vi "qODC.vi"(0 "System no.":i32=1 min=1 max=4 step=1, 2 "Axes to query":string[](array[string]), 3 "All axes?":bool, 4 "Axis identifier?":bool=TRUE, 5 "error in":errorcluster) -> (14 "Deceleration":dbl[](array[numeric]) format="%.6f", 19 "error out":errorcluster)   [LabVIEW 2020]
doc: "Returns open-loop deceleration setting for specified axes.\n\nE-861, E-874: If All axes? = TRUE, then Axis identifier? can be FALSE. Deceleration unit is steps/s²."
panel:
  # "Returns open-loop deceleration setting for specified axes."
  # "If all axes: use"
  # "Query"
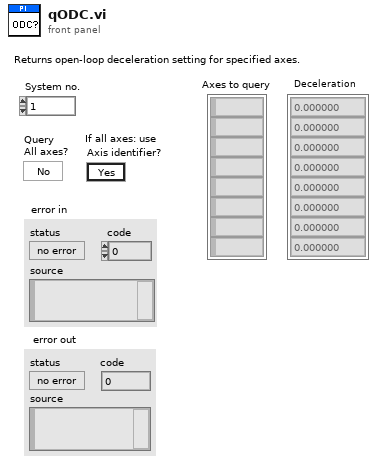
[diagram p1: front panel]
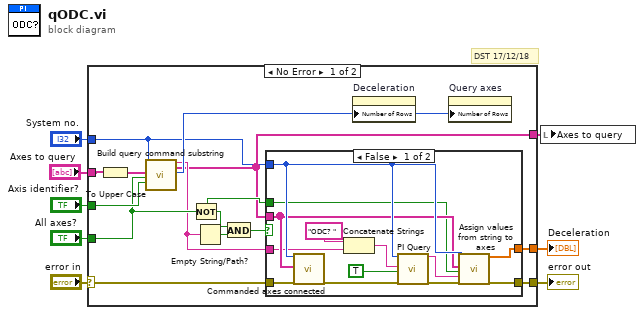
[diagram p0: block diagram]
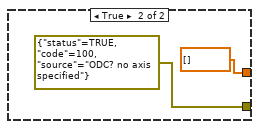
[diagram p2: hidden frame]
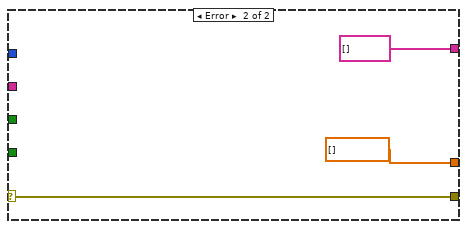
[diagram p3: hidden frame]
diagram:
  # "DST 17/12/18"
  n1 = case shown="No Error" "error in" {
    selector: "error in" -> [w10 w38]
    tunnel: [w22 dbl[] [] ("Values")] -> w8
    tunnel: "Axes to query" -> [w21 _]
    tunnel: [w20 w38] -> w6
    tunnel: "Axis identifier?" -> [w18 _]
    tunnel: "System no." -> [w16 _]
    tunnel: "All axes?" -> [w15 _]
    tunnel: [w9 string[] [] ("Axes to query out")] -> w1
    frame No Error {
      n2 = To Upper Case(1:w21) -> (0:w19:string[])
      n3 = call "Build query command substring.vi"("System no."=w16, "Axes to query in"=w19, "Query\nAll axes?"=w15, "For all axes: use\nAxis identifier?"=w18) -> ("Command substring"=w13:string, "Axes to query out"=w9:string[], "Number of rows"=w17:u32)  [unwired: 2 in, 11 out]
      n4 = Not(x=w15) -> (.not. x?=w14:bool)
      n5 = Empty String/Path?(string/path=w13) -> (empty?=w12:bool)
      n6 = And(x=w14, y=w12) -> (x .and. y?=w11:bool)
      n7 = case shown="False" w11 {
        tunnel: [w32 dbl[] [] ("Values")] -> w22
        tunnel: w10 -> [w31 _]
        tunnel: [w27 errorcluster {"status"=TRUE, "code"=100, "source"="ODC? no axis specified"} ("error out")] -> w20
        tunnel: w16 -> [w30 _]
        tunnel: w9 -> [w29 _]
        tunnel: w15 -> [w28 _]
        tunnel: w13 -> [w23 _]
        frame False {
          n8 = call "Commanded axes connected.vi"("System no."=w30, "Commanded axes"=w29, "error in"=w31) -> ("error out"=w26:errorcluster)  [unwired: 1 in, 15 out]
          n9 = Concatenate Strings("ODC? ", w23) -> (w33:string)
          n10 = call "PI Query.vi"("System no."=w30, "String to send"=w33, "Attach termination char.?"=TRUE ("Attach Linefeed?"), "error in"=w26) -> ("String read"=w25:string, "error out"=w24:errorcluster)  [unwired: 3 in, 11 out]
          n11 = call "Assign values from string to axes.vi"("System no."=w30, "Queried axes"=w29, "All axes queried?"=w28, "Input String"=w25, "error in"=w24) -> ("Values"=w32:dbl[], "error out"=w27:errorcluster)  [unwired: 4 in, 9 out]
        }
        frame True {
        }
      }
      n12 = property on="Deceleration" class="Arr (strict)"("Number of Rows"=w17) -> ()  [unwired: 2 in, 2 out]
      n13 = property on="Query axes" class="Arr (strict)"("Number of Rows"=w17) -> ()  [unwired: 2 in, 2 out]
    }
    frame Error {
    }
  }
  "error out" <- w6
  "Deceleration" <- w8
  n14 = local write "Axes to query"(w1) -> ()
